vi "Configure Trigger (Pattern).vi"(0 "VISA resource name":refnum<visa-resource-name>, 1 "Channel Settings":T1={"Channel 1 Input Setting"=2, "Channel 2 Input Setting"=2, "Channel 3 Input Setting"=2, "Channel 4 Input Setting"=2, "External  Input Setting"=2} {"External  Input Setting" items=["Low", "High", "X"]; "Channel 4 Input Setting" items=["Low", "High", "X"]; "Channel 3 Input Setting" items=["Low", "High", "X"]; "Channel 2 Input Setting" items=["Low", "High", "X"]; "Channel 1 Input Setting" items=["Low", "High", "X"]}, 2 "External Input Trigger Source (0: External)":u16(ring) items=["External", "External5"], 5 "Trigger Source (1: Channel 1)":u16(ring)=1 items=["Channel 1"=1, "Channel 2"=2, "Channel 3"=3, "Channel 4"=4, "External"=5, "External 5"=6], 7 "Trigger Modifier (0: Auto)":u16(ring) items=["Auto", "Normal", "Single"], 9 "Trigger Level (0.0 V)":dbl, 11 "error in (no error)":errorcluster, 12 "Edge Source (0: Channel 1)":u16(ring) items=["Channel 1", "Channel 2", "Channel 3", "Channel 4", "External", "External 5"], 13 "Edge Direction (1: Positive)":u16(ring)=1 items=["Negative", "Positive"], 14 "Enable Edge Trigger (F: Disable)":bool) -> (4 "VISA resource name out":refnum<visa-resource-name>, 15 "error out":errorcluster)   [LabVIEW 2010, in "Agilent DSO1000 Series.lvlib"]
doc: "Configures pattern trigger settings.You define the pattern by setting the <B>Channel Settings</B>. If you enable the edge trigger, set <B>Edge Source</B> and <B>Edge Dir</B> value."
uses:
  <instrlib>/Agilent DSO1000 Series/Agilent DSO1000 Series.lvlib
panel:
  # "Input Edge Trigger Setting"
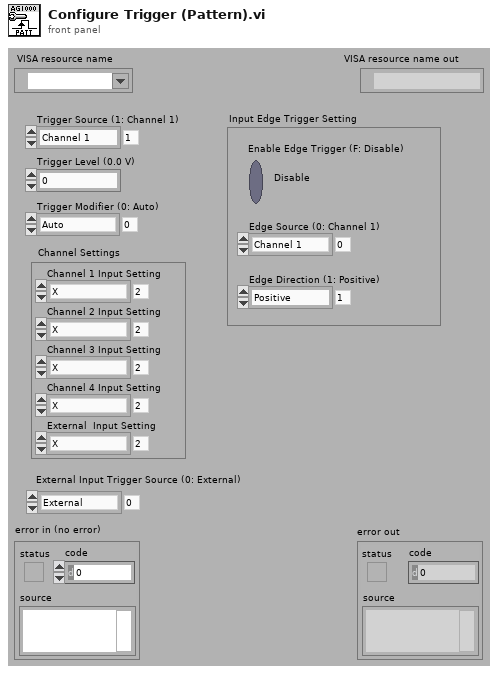
[diagram p1: front panel]
types:
  T1 = cluster{"Channel 1 Input Setting":u16, "Channel 2 Input Setting":u16, "Channel 3 Input Setting":u16, "Channel 4 Input Setting":u16, "External  Input Setting":u16}
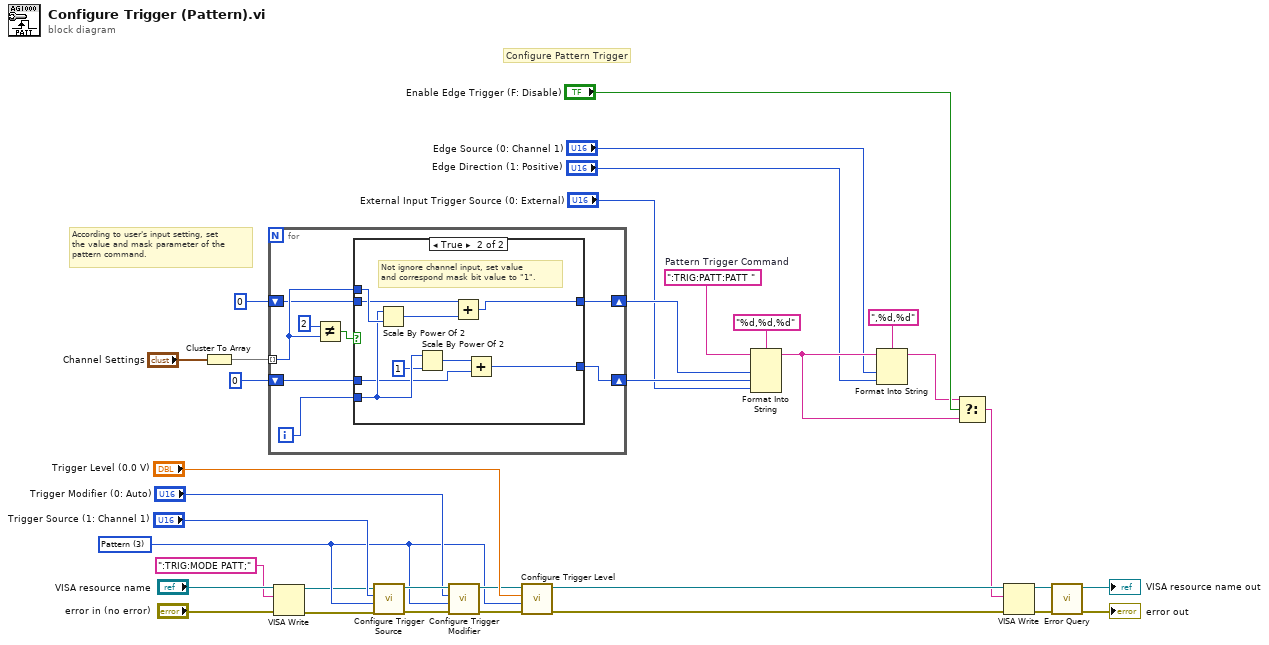
[diagram p0: block diagram]
diagram:
  w6 = u16 3 items=["Edge", "Pulse", "TV", "Pattern"] ("Trigger Type")
  w16 = ":TRIG:PATT:PATT "  # Pattern Trigger Command
  # "According to user's input setting, set \nthe value and mask parameter of the\npattern command."
  # "Configure Pattern Trigger"
  n1 = Cluster To Array(cluster="Channel Settings") -> (array=w23:u16[])
  n2 = for {
    tunnel: w23 -> [w42] mode=indexing
    shift-right: [w41] -> w17
    shift-left: 0 -> [w38]
    shift-right: [w37] -> w18
    shift-left: 0 -> [w39]
    i -> [w36]
    n3 = Not Equal?(x=2, y=w42) -> (x != y?=w43:bool)
    n4 = case shown="True" w43 {
      tunnel: w42 -> [_ w54]
      tunnel: w36 -> [_ w53]
      tunnel: [w45 w49] -> w41
      tunnel: w39 -> [w44 w47]
      tunnel: w38 -> [w45 w50]
      tunnel: [w44 w48] -> w37
      frame False {
        # "Ignore channel input"
      }
      frame True {
        # "Not ignore channel input, set value\nand correspond mask bit value to \"1\"."
        n5 = Scale By Power Of 2(n=w53, x=w54) -> (x*2^n=w46:u16)
        n6 = Scale By Power Of 2(n=w53, x=1) -> (x*2^n=w51:i32)
        n7 = Add(x=w47, y=w46) -> (x+y=w48:i32)
        n8 = Add(x=w51, y=w50) -> (x+y=w49:i32)
      }
    }
  }
  n9 = VISA Write(VISA resource name="VISA resource name", write buffer=":TRIG:MODE PATT;", error in (no error)="error in (no error)") -> (VISA resource name out=w3:refnum<visa-resource-name>, error out=w2:errorcluster)  [unwired: 1 out]
  n10 = call <instrlib>:"Configure Trigger Source.vi"("error in (no error)"=w2, "Trigger Type"=w6, "Trigger Source (1: Channel 1)"="Trigger Source (1: Channel 1)", "VISA resource name"=w3) -> ("error out"=w31:errorcluster, "VISA resource name out"=w30:refnum<visa-resource-name>)  [unwired: 6 in]
  n11 = call <instrlib>:"Configure Trigger Modifier.vi"("error in (no error)"=w31, "Trigger Type"=w6, "Trigger Modifier (0: Auto)"="Trigger Modifier (0: Auto)", "VISA resource name"=w30) -> ("error out"=w26:errorcluster, "VISA resource name out"=w27:refnum<visa-resource-name>)  [unwired: 6 in]
  n12 = call <instrlib>:"Configure Trigger Level.vi"("error in (no error)"=w26, "Trigger Type"=w6, "Trigger Level (0.0 V)"="Trigger Level (0.0 V)", "VISA resource name"=w27) -> ("error out"=w19:errorcluster, "VISA resource name out"=w20:refnum<visa-resource-name>)  [unwired: 6 in]
  n13 = Format Into String(format string="%d,%d,%d", initial string=w16, w18, w17, "External Input Trigger Source (0: External)") -> (resulting string=w10:string)  [unwired: 1 in, 1 out]
  n14 = Format Into String(format string=",%d,%d", initial string=w10, "Edge Source (0: Channel 1)", "Edge Direction (1: Positive)") -> (resulting string=w11:string)  [unwired: 1 in, 1 out]
  n15 = Select(t=w11, s="Enable Edge Trigger (F: Disable)", f=w10) -> (s? t:f=w9:string)
  n16 = VISA Write(VISA resource name=w20, write buffer=w9, error in (no error)=w19) -> (VISA resource name out=w33:refnum<visa-resource-name>, error out=w32:errorcluster)  [unwired: 1 out]
  n17 = call <instrlib>:"Error Query.vi"("error in (no error)"=w32, "VISA resource name"=w33) -> ("error out"=→"error out":errorcluster, "VISA resource name out"=→"VISA resource name out":refnum<visa-resource-name>)  [unwired: 6 in, 2 out]
